vi "To Gray_FPGA (SubVI).vi"(6 "Pixel Data":cluster{"A":u8, "R/H":u8, "G/S":u8, "B/L":u8}, 9 "DV":bool, 10 "EOL":bool, 11 "EOI":bool) -> (3 "Pixel Bus In":T1)   [LabVIEW 2016]
uses:
  <vilib>/visionFPGA/Controls/IMAQ FPGA Pixel Bus u8x1.ctl
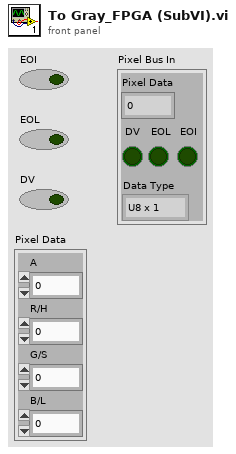
[diagram p1: front panel]
types:
  T1 = typedef "IMAQ FPGA Pixel Bus u8x1.ctl" = cluster{"Pixel Data":u8, "DV":bool, "EOL":bool, "EOI":bool, "Data Type":enum16{"U8 x 1"}}
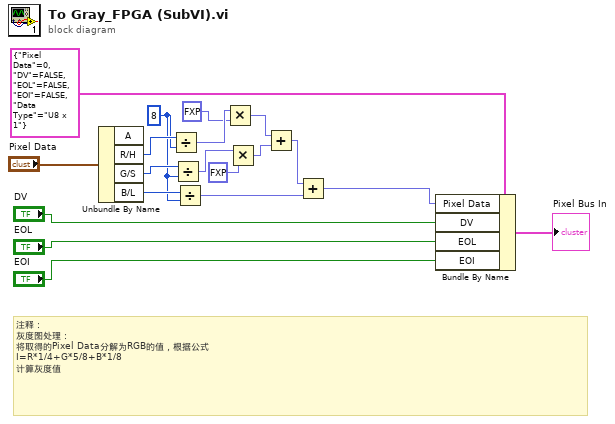
[diagram p0: block diagram]
diagram:
  w10 = u8 8 ("y")
  # "注释：\n灰度图处理：\n将取得的Pixel Data分解为RGB的值，根据公式\nI=R*1/4+G*5/8+B*1/8\n计算灰度值"
  n1 = Unbundle By Name("Pixel Data") -> ("R/H"=w13:u8, "G/S"=w12:u8, "B/L"=w11:u8)  [unwired: 1 out]
  n2 = Divide(x=w13, y=w10) -> (x/y=w9:fxp<+,8,26>)
  n3 = Divide(x=w12, y=w10) -> (x/y=w7:fxp<+/-,32,26>)
  n4 = Divide(x=w11, y=w10) -> (x/y=w2:fxp<+/-,32,26>)
  n5 = Multiply(x=w9, y=fxp<+/-,32,26> 2.0) -> (x*y=w5:fxp<+/-,40,52>)
  n6 = Multiply(x=w7, y=fxp<+/-,32,26> 5.0) -> (x*y=w4:fxp<+/-,64,52>)
  n7 = Add(x=w5, y=w4) -> (x+y=w3:fxp<+/-,64,53>)
  n8 = Add(x=w3, y=w2) -> (x+y=w1:fxp<+/-,64,54>)
  n9 = Bundle By Name(cluster=T1 {"Pixel Data"=0, "DV"=FALSE, "EOL"=FALSE, "EOI"=FALSE, "Data Type"=enum."U8 x 1"} ("Pixel Bus In"), "Pixel Data"=w1, "DV"="DV", "EOL"="EOL", "EOI"="EOI") -> (→"Pixel Bus In":T1)
